vi "Return Default Object.vi"(11 "Object":refnum<class>) -> (2 "Object (default)":refnum<class>, 3 "Object (duplicate)":refnum<class>)   [LabVIEW 2021]
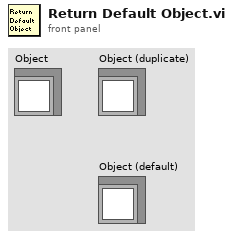
[diagram p1: front panel]
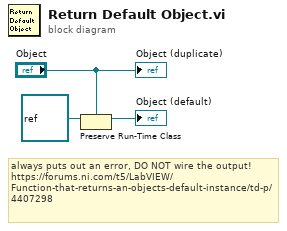
[diagram p0: block diagram]
diagram:
  # "always puts out an error, DO NOT wire the output!\nhttps://forums.ni.com/t5/LabVIEW/Function-that-returns-an-objects-default-instance/td-p/4407298"
  n1 = Preserve Run-Time Class(object in=refnum<class> refnum ("LabVIEW Object"), 2:"Object") -> (object out=→"Object (default)":refnum<class>)  [unwired: 1 in, 1 out]
  "Object (duplicate)" <- "Object"
